vi "p1 solution.vi"(11 "Dir List":cluster{"Name":string, "Size":i64}[](array[cluster])) -> (3 "Size":i64)   [LabVIEW 2021, in "d7.lvlib"]
uses:
  d7.lvlib
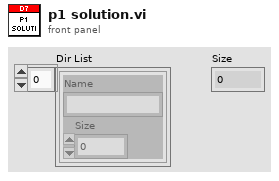
[diagram p1: front panel]
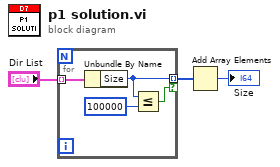
[diagram p0: block diagram]
diagram:
  n1 = for {
    tunnel: "Dir List" -> [w7] mode=indexing
    tunnel: [w5] -> w2 mode=indexing if=w4
    n2 = Unbundle By Name(w7) -> ("Size"=w5:i64)
    n3 = Less Or Equal?(x=w5, y=i64 100000) -> (x <= y?=w4:bool)
  }
  n4 = Add Array Elements(numeric array=w2) -> (sum=→"Size":i64)
